vi "ClientLabView_VictorV3.vi"() -> ()   [LabVIEW 2014]
panel:
  in  "Nombre de mostres mitjana":u32=1 min=1 max=9 step=1
  in  "Temps de mostratge":u32=1 min=1 max=20 step=1
  in  "Missatge a enviar":string(combo)="No enviar res"
  out "String":string
  out "Mostres Guardades":string
  out "Reset":string
  out "Status":string
  out "Temperatura Mínima":string
  out "Temperatura Màxima":string
  out "Mostra més antiga":string
  in  "Port":i32=5001
  in  "IP Adress":string="192.168.0.181"
  in  "?":bool
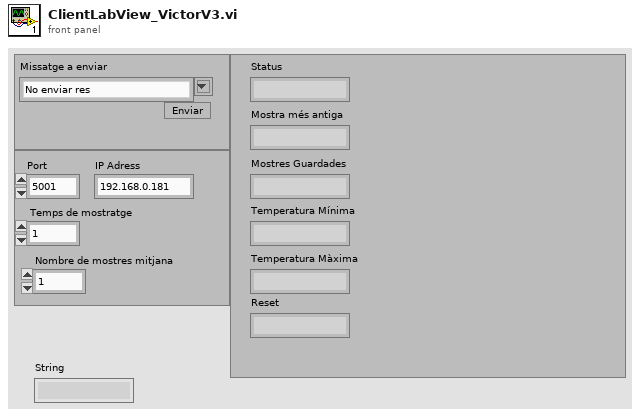
[diagram p1: front panel]
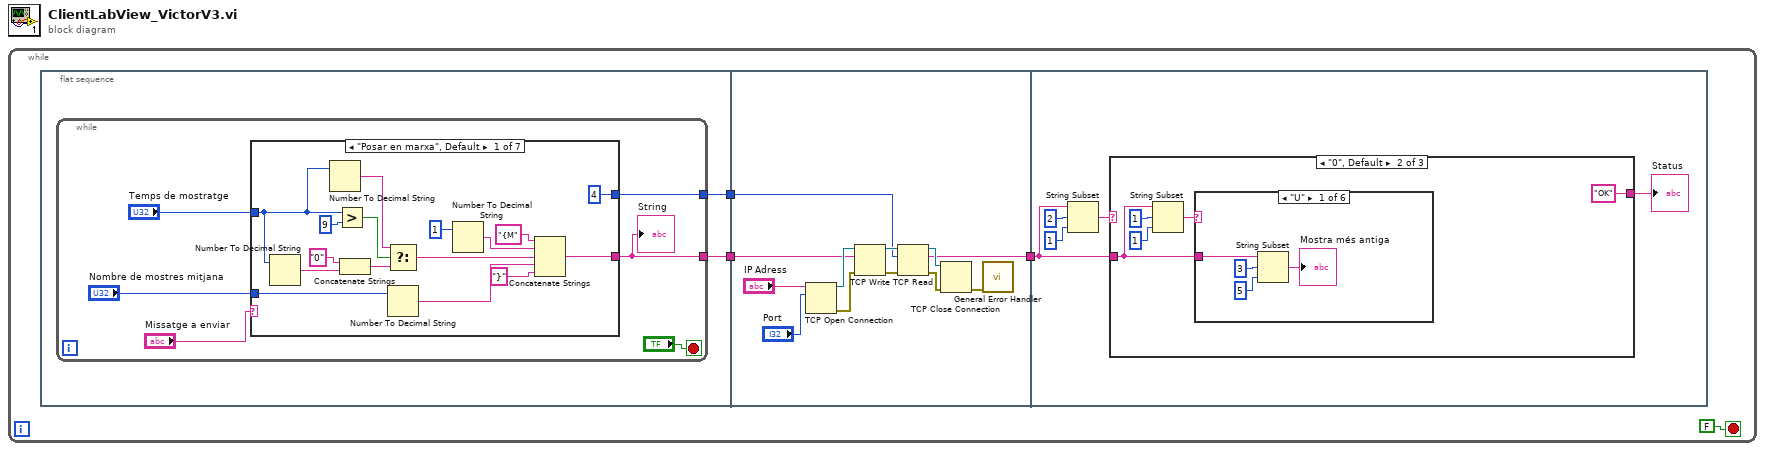
[diagram p0: block diagram]
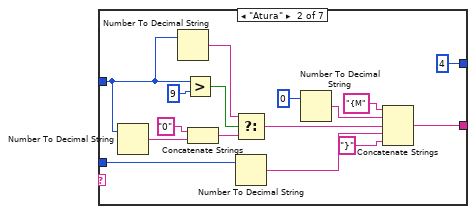
[diagram p2: hidden frame]
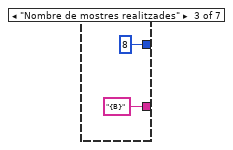
[diagram p3: hidden frame]
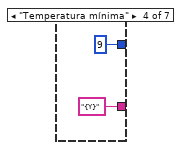
[diagram p4: hidden frame]
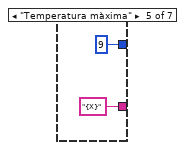
[diagram p5: hidden frame]
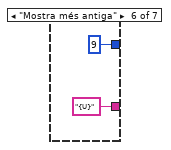
[diagram p6: hidden frame]
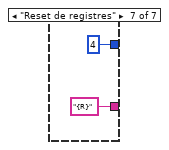
[diagram p7: hidden frame]
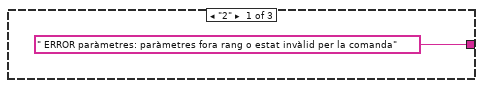
[diagram p8: hidden frame]
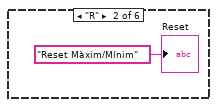
[diagram p9: hidden frame]
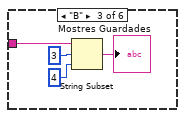
[diagram p10: hidden frame]
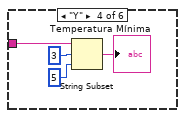
[diagram p11: hidden frame]
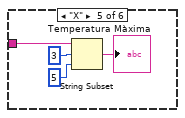
[diagram p12: hidden frame]
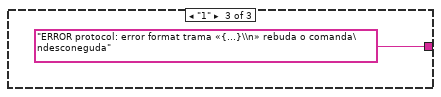
[diagram p14: hidden frame]
diagram:
  n1 = while {
    stop <- FALSE stop-if-true
    n2 = flat-sequence {
      tunnel: [w6] -> w2
      tunnel: [w5] -> w1
      tunnel: [w57] -> w3
      tunnel: w2 -> [w56]
      tunnel: w1 -> [w55]
      tunnel: w3 -> [w68]
      frame #0 {
        n3 = while {
          tunnel: [w7] -> w6
          tunnel: [w8] -> w5
          stop <- "?" stop-if-true
          n4 = case shown="\"Posar en marxa\", Default" "Missatge a enviar" {
            tunnel: [w20 w29 "{B}" "{Y}" "{X}" "{U}" "{R}"] -> w7
            tunnel: [4 4 8 9 9 9 4] -> w8
            tunnel: "Temps de mostratge" -> [w21 w37 _ _ _ _ _]
            tunnel: "Nombre de mostres mitjana" -> [w15 w33 _ _ _ _ _]
            frame "Posar en marxa", Default {
              n5 = Number To Decimal String(number=w21) -> (decimal integer string=w25:string)  [unwired: 1 in]
              n6 = Number To Decimal String(number=w21) -> (decimal integer string=w23:string)  [unwired: 1 in]
              n7 = Greater?(x=w21, y=u32 9) -> (0:w27:bool)
              n8 = Concatenate Strings("0" ("string"), w25) -> (w24:string)
              n9 = Select(t=w23, s=w27, f=w24) -> (s? t:f=w16:string)
              n10 = Number To Decimal String(number=w15) -> (decimal integer string=w14:string)  [unwired: 1 in]
              n11 = Number To Decimal String(number=1 ("input 3")) -> (decimal integer string=w17:string)  [unwired: 1 in]
              n12 = Concatenate Strings("{M", w17, w16, w14, "}") -> (w20:string)
            }
            frame "Atura" {
              n13 = Number To Decimal String(number=w37) -> (decimal integer string=w41:string)  [unwired: 1 in]
              n14 = Number To Decimal String(number=w37) -> (decimal integer string=w39:string)  [unwired: 1 in]
              n15 = Greater?(x=w37, y=u32 9) -> (0:w43:bool)
              n16 = Concatenate Strings("0" ("string"), w41) -> (w40:string)
              n17 = Select(t=w39, s=w43, f=w40) -> (s? t:f=w30:string)
              n18 = Number To Decimal String(number=w33) -> (decimal integer string=w35:string)  [unwired: 1 in]
              n19 = Number To Decimal String(number=0 ("input 3")) -> (decimal integer string=w31:string)  [unwired: 1 in]
              n20 = Concatenate Strings("{M", w31, w30, w35, "}") -> (w29:string)
            }
            frame "Nombre de mostres realitzades" {
            }
            frame "Temperatura mínima" {
            }
            frame "Temperatura màxima" {
            }
            frame "Mostra més antiga" {
            }
            frame "Reset de registres" {
            }
          }
          "String" <- w7
        }
      }
      frame #1 {
        n21 = TCP Open Connection(address="IP Adress", remote port or service name="Port") -> (connection ID=w64:refnum<k5>, error out=w61:errorcluster)  [unwired: 3 in]
        n22 = TCP Write(connection ID=w64, data in=w56, error in (no error)=w61) -> (connection ID out=w65:refnum<k5>, error out=w60:errorcluster)  [unwired: 1 in, 1 out]
        n23 = TCP Read(connection ID=w65, bytes to read=w55, error in (no error)=w60) -> (connection ID out=w66:refnum<k5>, data out=w57:string, error out=w59:errorcluster)  [unwired: 2 in]
        n24 = TCP Close Connection(connection ID=w66, error in (no error)=w59) -> (error out=w58:errorcluster)  [unwired: 1 in, 1 out]
        n25 = call <vilib>:"General Error Handler.vi"("error in (no error)"=w58) -> ()  [unwired: 10 in, 5 out]
      }
      frame #2 {
        n26 = String Subset(string=w68, offset (0)=2, length (rest)=1 ("length (rest)")) -> (substring=w71:string)
        n27 = case shown="\"0\", Default" w71 {
          tunnel: w68 -> [_ w74 _]
          tunnel: [" ERROR paràmetres: paràmetres fora rang o estat invàlid per la comanda" "OK" "ERROR protocol: error format trama «{...}\\n» rebuda o comanda\ndesconeguda"] -> w67
          frame "2" {
          }
          frame "0", Default {
            n28 = String Subset(string=w74, offset (0)=1, length (rest)=1 ("length (rest)")) -> (substring=w75:string)
            n29 = case shown="\"U\"" w75 {
              tunnel: w74 -> [w81 _ w83 w87 w91 _]
              frame "U" {
                n30 = String Subset(string=w81, offset (0)=3, length (rest)=5 ("length (rest)")) -> (substring=→"Mostra més antiga":string)
              }
              frame "R" {
                "Reset" <- "Reset Màxim/Mínim"
              }
              frame "B" {
                n31 = String Subset(string=w83, offset (0)=3, length (rest)=4 ("length (rest)")) -> (substring=→"Mostres Guardades":string)
              }
              frame "Y" {
                n32 = String Subset(string=w87, offset (0)=3, length (rest)=5 ("length (rest)")) -> (substring=→"Temperatura Mínima":string)
              }
              frame "X" {
                n33 = String Subset(string=w91, offset (0)=3, length (rest)=5 ("length (rest)")) -> (substring=→"Temperatura Màxima":string)
              }
              frame "M", Default {
              }
            }
          }
          frame "1" {
          }
        }
        "Status" <- w67
      }
    }
  }
